vi "Check Closed Loop.vi"(9 "Answer":i32, 10 "Str Refnum":refnum<vi>, 11 "Digital in":refnum<vi>) -> (2 "Bit 0":bool)   [LabVIEW 2021]
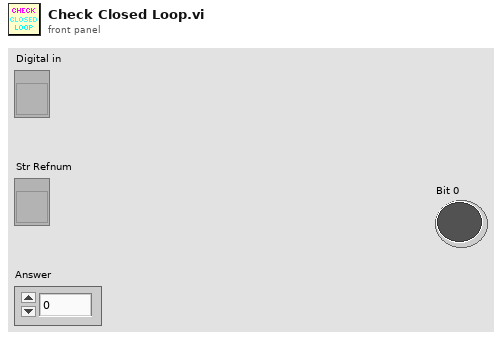
[diagram p1: front panel]
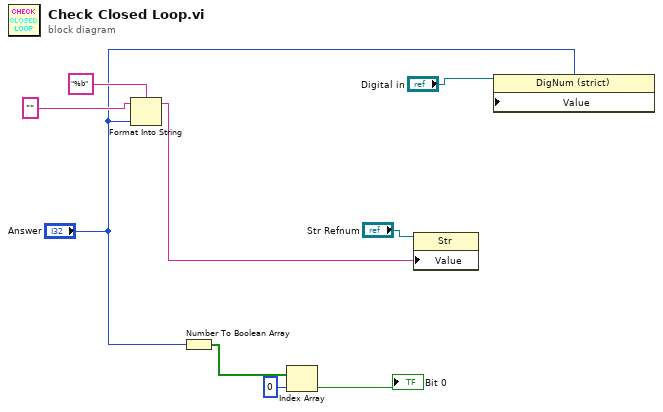
[diagram p0: block diagram]
diagram:
  n1 = Format Into String(format string="%b" ("initial string"), initial string="", "Answer") -> (resulting string=w7:string)  [unwired: 1 in, 1 out]
  n2 = Number To Boolean Array(number="Answer") -> (Boolean array=w3:bool[])
  n3 = Index Array(array=w3, index=0) -> (element=→"Bit 0":bool)
  n4 = property on="Property Node" class="Str"(reference="Str Refnum", "Value"=w7) -> ()  [unwired: 1 in, 2 out]
  n5 = property on="Property Node" class="DigNum (strict)"(reference="Digital in", "Value"="Answer") -> ()  [unwired: 1 in, 2 out]
